vi "To-do-list-Labview.vi"() -> ()   [LabVIEW 2022 SP3]
uses:
  <vilib>/addons/database/Connection.llb/DB Tools Open Connec (String).vi
  <vilib>/addons/database/Connection.llb/Conn Execute.vi
  <vilib>/addons/database/Recordset.llb/Rec Destroy - Connection.vi
  <vilib>/addons/database/NI_Database_API.lvlib
panel:
  in  "TOT":bool
  in  "Afisare":bool
  in  "Calendar":timestamp=timestamp(3755242155.0327334 s since 1904-01-01) format="%<%x>T"
  in  "Efectuat":bool
  in  "Actualizare":bool
  in  "Stergere":bool
  in  "Editare":string
  in  "Sarcina de inserat":string
  in  "Inserare":bool
  in  "Alege linia":u16(ring) items=["1", "2", "4", "5", "9", "10", "11", "12", "14", "15", "16", "17"]
  out "Linii":i32
  out "Coloane":i32
  out "Lista de sarcini":string[][](table)
  # "Proiectul de fata are scopul de a facilita utilizatorului o metoda de a stoca, citii, edita, sterge informatii pe care le doreste. \n    Cu alte cuvinte, proiectul este un ToDoList in care, cu operatii de tip CRUD, se pot accesa datele dintr-o baza de date, iar utilizatorul are acces total la informatiile pe care acesta le introduce.\n     Ca si baza de date am ales Microsoft MySQL ce permite cu usurinta administratorilor sa acceseze datele in baze de date."
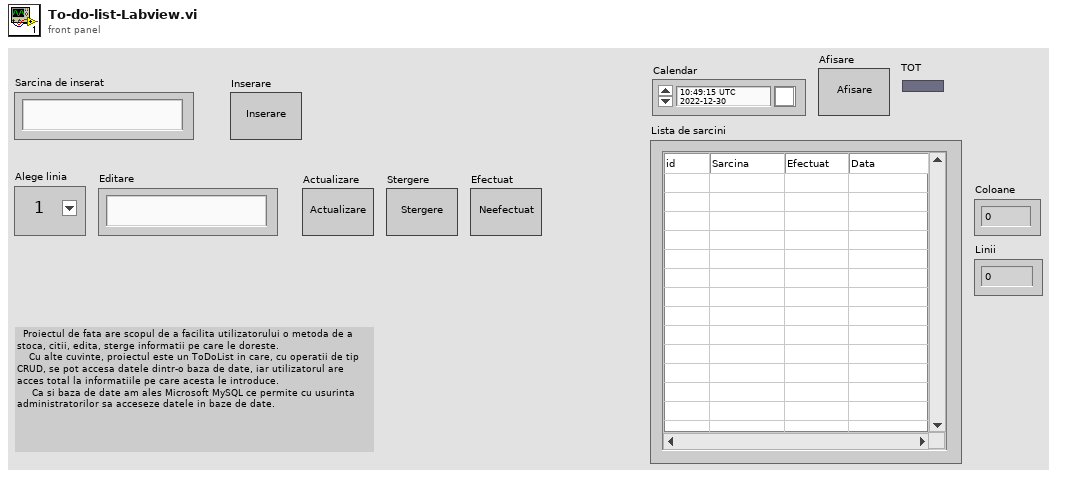
[diagram p1: front panel]
types:
  T1 = typedef "NI_Database_API.lvlib/Conn ObjectReference.ctl" = refnum<k1>
  T2 = typedef "NI_Database_API.lvlib/Rec ObjectReference.ctl" = refnum<k1>
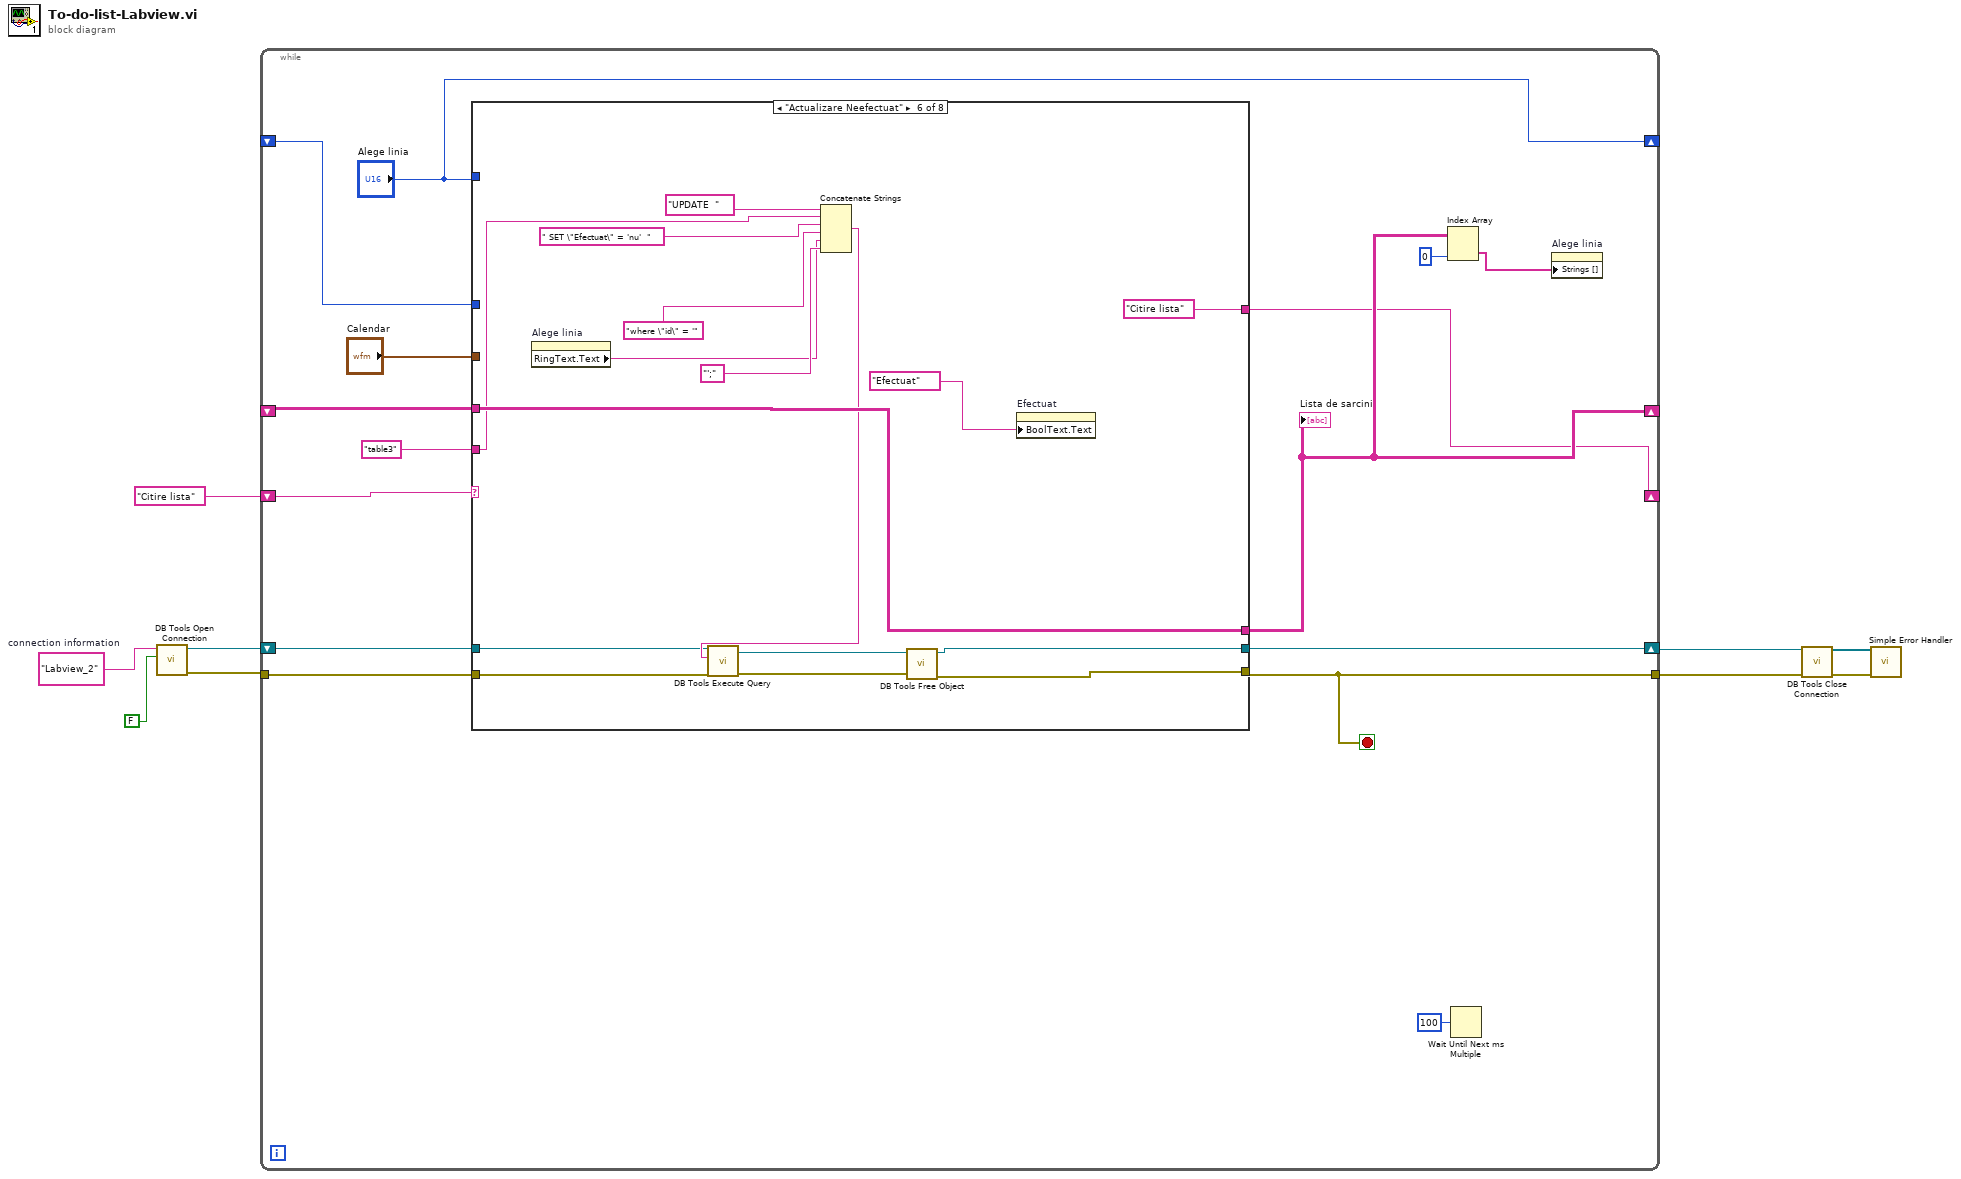
[diagram p0: block diagram]
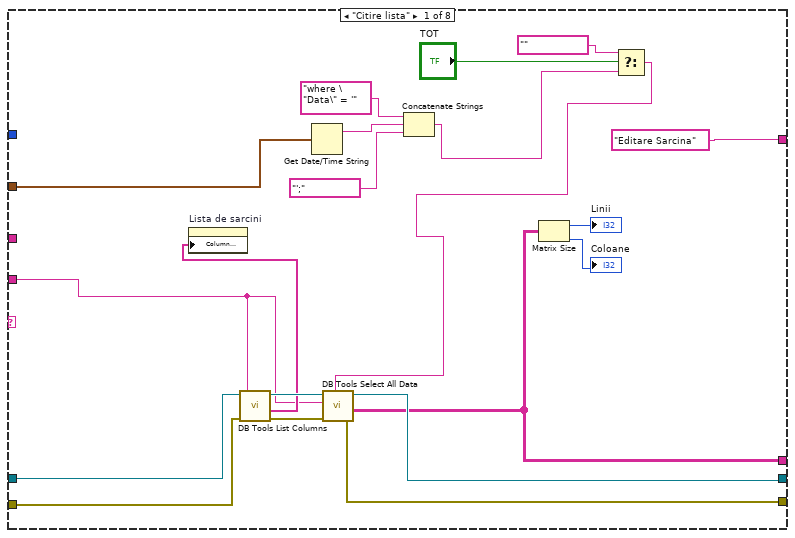
[diagram p2: hidden frame]
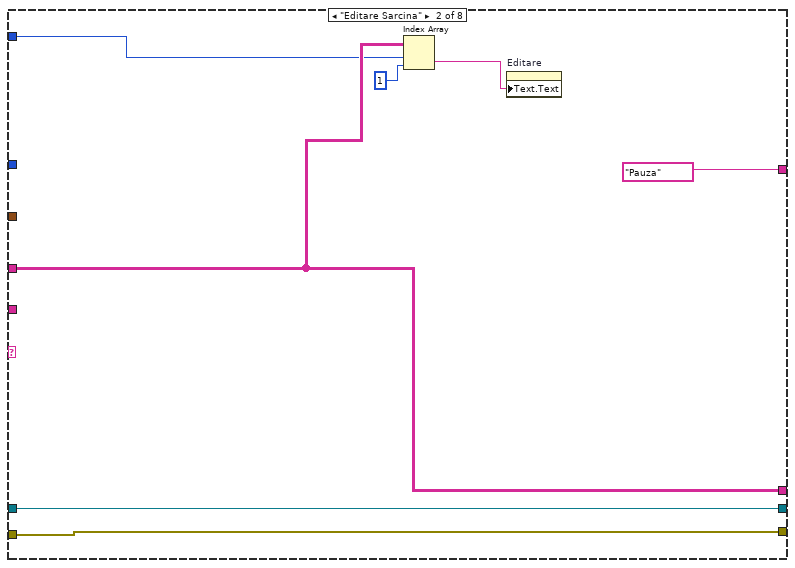
[diagram p3: hidden frame]
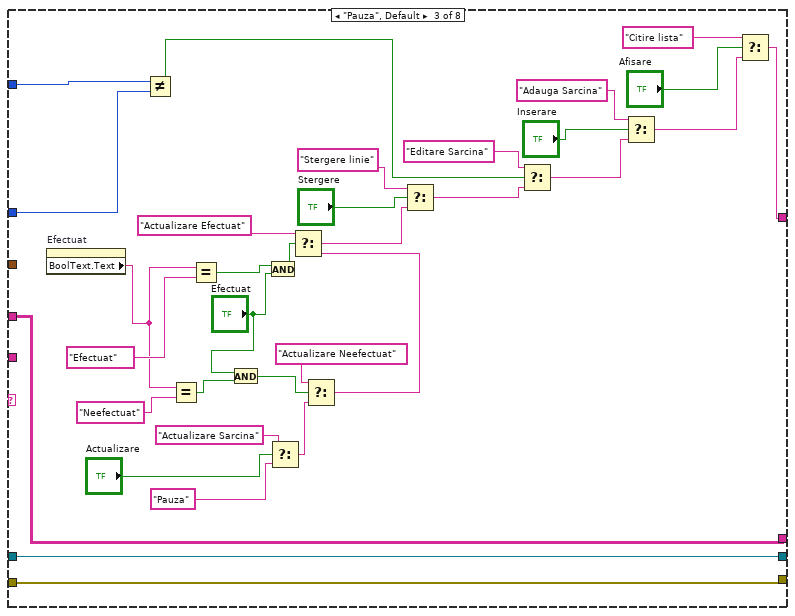
[diagram p4: hidden frame]
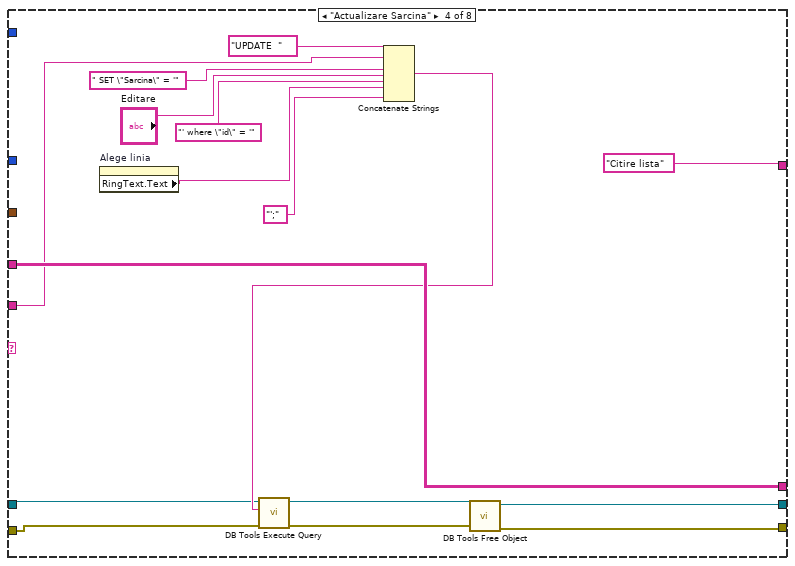
[diagram p5: hidden frame]
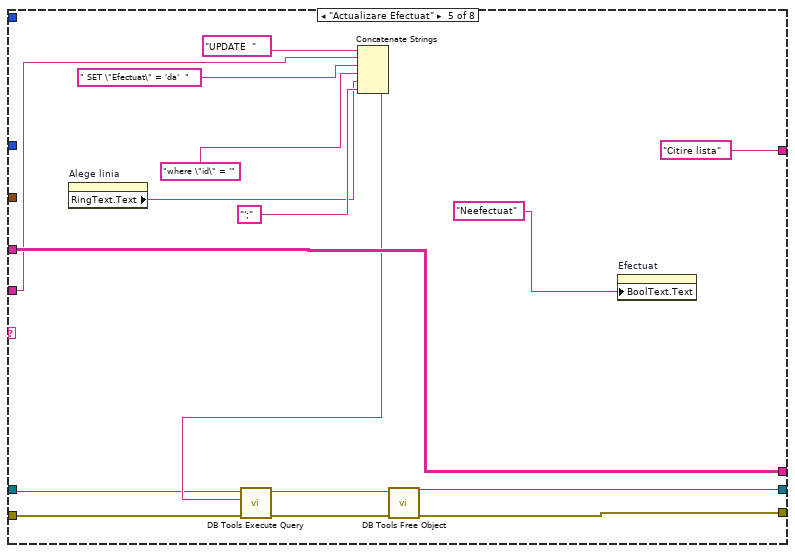
[diagram p6: hidden frame]
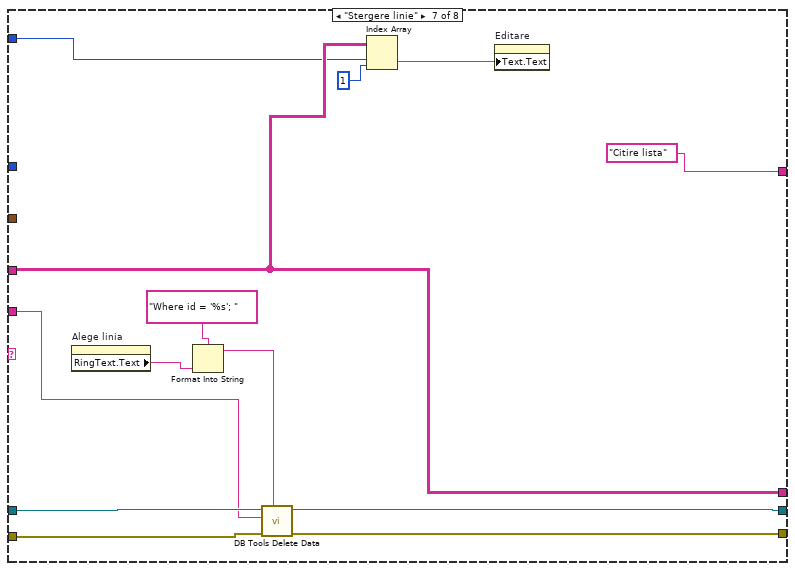
[diagram p7: hidden frame]
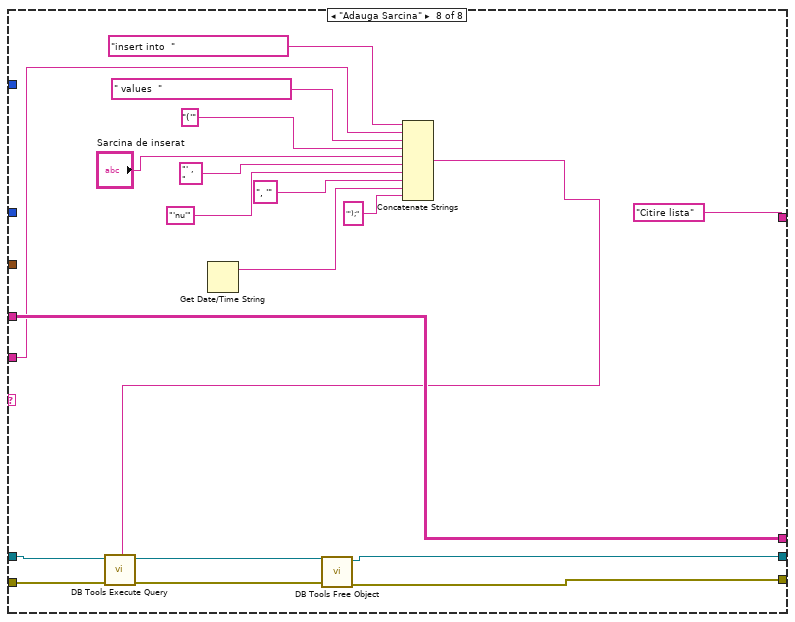
[diagram p8: hidden frame]
diagram:
  w8 = "Labview_2"  # connection information
  n1 = call-poly <vilib>:"DB Tools Open Connection.vi"("prompt? (F)"=FALSE, "connection information"=w8) -> ("error out"=w6:errorcluster, "connection reference"=w7:T1)  [unwired: 6 in]
  n2 = while {
    shift-right: [w20] -> w3
    shift-left: w7 -> [w22]
    tunnel: w6 -> [w23]
    tunnel: [w21] -> w4
    shift-right: [w9] -> _
    shift-left: "Citire lista" -> [w19]
    shift-right: [w14] -> _
    shift-left: _ -> [w17]
    shift-right: ["Alege linia"] -> _
    shift-left: _ -> [w12]
    stop <- w21 stop-if-true
    n3 = case shown="\"Actualizare Neefectuat\"" w19 {
      tunnel: w23 -> [w35 w49 w80 w86 w106 w121 w141 w161]
      tunnel: w22 -> [w37 w50 w81 w89 w104 w117 w143 w148]
      tunnel: [w41 w49 w80 w84 w102 w119 w140 w145] -> w21
      tunnel: [w40 w50 w81 w87 w100 w116 w142 w147] -> w20
      tunnel: ["Editare Sarcina" "Pauza" w82 "Citire lista" "Citire lista" "Citire lista" "Citire lista" "Citire lista"] -> w9
      tunnel: [w38 w46 w79 w98 w114 w130 w135 w162] -> w14
      tunnel: w17 -> [_ w46 w79 w98 w114 w130 w135 w162]
      tunnel: "Alege linia" -> [_ w44 w74 _ _ _ w134 _]
      tunnel: w12 -> [_ _ w73 _ _ _ _ _]
      tunnel: "table3" ("table") -> [w32 _ _ w96 w112 w128 w132 w151]
      tunnel: "Calendar" -> [w31 _ _ _ _ _ _ _]
      frame "Citire lista" {
        n4 = call <vilib>:"DB Tools List Columns.vi"("error in (no error)"=w35, "table"=w32, "connection reference"=w37) -> ("error out"=w34:errorcluster, "columns"=w33:string[], "connection reference out"=w36:T1)  [unwired: 1 in, 1 out]
        n5 = property on="Lista de sarcini" class="Tbl (strict)"("Column Headers[]"=w33) -> ()  [unwired: 2 in, 2 out]
        n6 = Get Date/Time String(seconds (now)=w31) -> (date string=w29:string)  [unwired: 2 in, 1 out]
        n7 = Concatenate Strings("where \"Data\" = '", w29, "';") -> (w25:string)
        n8 = Select(t="", s="TOT", f=w25) -> (s? t:f=w27:string)
        n9 = call <vilib>:"DB Tools Select All Data.vi"("optional clause"=w27, "error in (no error)"=w34, "table"=w32, "connection reference"=w36) -> ("error out"=w41:errorcluster, "data"=w38:string[][], "connection reference out"=w40:T1)  [unwired: 2 in]
        n10 = Matrix Size(0:w38) -> (1:→"Linii":i32, 2:→"Coloane":i32)
      }
      frame "Editare Sarcina" {
        n11 = Index Array(array=w46, index (row)=w44, index (col)=1) -> (element=w45:string)
        n12 = property on="Editare" class="Str"("Text.Text"=w45) -> ()  [unwired: 2 in, 2 out]
      }
      frame "Pauza", Default {
        n13 = property on="Efectuat" class="Bool"() -> ("BoolText.Text"=w63:string)  [unwired: 2 in, 2 out]
        n14 = Not Equal?(x=w74, y=w73) -> (x != y?=w72:bool)
        n15 = Equal?(x=w63, y="Neefectuat") -> (x = y?=w56:bool)
        n16 = Equal?(x=w63, y="Efectuat") -> (x = y?=w59:bool)
        n17 = And(x="Efectuat", y=w56) -> (x .and. y?=w55:bool)
        n18 = And(x=w59, y="Efectuat") -> (x .and. y?=w58:bool)
        n19 = Select(t="Actualizare Sarcina", s="Actualizare", f="Pauza") -> (s? t:f=w54:string)
        n20 = Select(t="Actualizare Neefectuat", s=w55, f=w54) -> (s? t:f=w61:string)
        n21 = Select(t="Actualizare Efectuat", s=w58, f=w61) -> (s? t:f=w66:string)
        n22 = Select(t="Stergere linie", s="Stergere", f=w66) -> (s? t:f=w65:string)
        n23 = Select(t="Editare Sarcina", s=w72, f=w65) -> (s? t:f=w76:string)
        n24 = Select(t="Adauga Sarcina", s="Inserare", f=w76) -> (s? t:f=w77:string)
        n25 = Select(t="Citire lista", s="Afisare", f=w77) -> (s? t:f=w82:string)
      }
      frame "Actualizare Sarcina" {
        n26 = property on="Alege linia" class="Ring (strict)"() -> ("RingText.Text"=w92:string)  [unwired: 2 in, 2 out]
        n27 = Concatenate Strings("UPDATE  " ("table"), w96, " SET \"Sarcina\" = '" ("table"), "Editare", "' where \"id\" = '" ("table"), w92, "';" ("table")) -> (w90:string)
        n28 = call-poly <vilib>:"DB Tools Execute Query.vi"("error in (no error)"=w86, "SQL query"=w90, "connection reference"=w89) -> ("error out"=w85:errorcluster, "recordset reference"=w88:T2)  [unwired: 5 in]
        n29 = call-poly <vilib>:"DB Tools Free Object.vi"("error in (no error)"=w85, "recordset reference"=w88) -> ("error out"=w84:errorcluster, "connection reference"=w87:T1)  [unwired: 8 in]
      }
      frame "Actualizare Efectuat" {
        n30 = property on="Alege linia" class="Ring (strict)"() -> ("RingText.Text"=w108:string)  [unwired: 2 in, 2 out]
        n31 = Concatenate Strings("UPDATE  " ("table"), w112, " SET \"Efectuat\" = 'da'  " ("table"), "where \"id\" = '" ("table"), w108, "';" ("table")) -> (w105:string)
        n32 = call-poly <vilib>:"DB Tools Execute Query.vi"("error in (no error)"=w106, "SQL query"=w105, "connection reference"=w104) -> ("error out"=w101:errorcluster, "recordset reference"=w103:T2)  [unwired: 5 in]
        n33 = call-poly <vilib>:"DB Tools Free Object.vi"("error in (no error)"=w101, "recordset reference"=w103) -> ("error out"=w102:errorcluster, "connection reference"=w100:T1)  [unwired: 8 in]
        n34 = property on="Efectuat" class="Bool"("BoolText.Text"="Neefectuat") -> ()  [unwired: 2 in, 2 out]
      }
      frame "Actualizare Neefectuat" {
        n35 = property on="Alege linia" class="Ring (strict)"() -> ("RingText.Text"=w123:string)  [unwired: 2 in, 2 out]
        n36 = Concatenate Strings("UPDATE  " ("table"), w128, " SET \"Efectuat\" = 'nu'  " ("table"), "where \"id\" = '" ("table"), w123, "';" ("table")) -> (w124:string)
        n37 = call-poly <vilib>:"DB Tools Execute Query.vi"("error in (no error)"=w121, "SQL query"=w124, "connection reference"=w117) -> ("error out"=w120:errorcluster, "recordset reference"=w118:T2)  [unwired: 5 in]
        n38 = call-poly <vilib>:"DB Tools Free Object.vi"("error in (no error)"=w120, "recordset reference"=w118) -> ("error out"=w119:errorcluster, "connection reference"=w116:T1)  [unwired: 8 in]
        n39 = property on="Efectuat" class="Bool"("BoolText.Text"="Efectuat") -> ()  [unwired: 2 in, 2 out]
      }
      frame "Stergere linie" {
        n40 = property on="Alege linia" class="Ring (strict)"() -> ("RingText.Text"=w139:string)  [unwired: 2 in, 2 out]
        n41 = Format Into String(format string="Where id = '%s'; " ("table"), w139) -> (resulting string=w137:string)  [unwired: 2 in, 1 out]
        n42 = call <vilib>:"DB Tools Delete Data.vi"("condition"=w137, "error in (no error)"=w141, "table"=w132, "connection reference"=w143) -> ("error out"=w140:errorcluster, "connection reference out"=w142:T1)  [unwired: 6 in]
        n43 = Index Array(array=w135, index (row)=w134, index (col)=1) -> (element=w133:string)
        n44 = property on="Editare" class="Str"("Text.Text"=w133) -> ()  [unwired: 2 in, 2 out]
      }
      frame "Adauga Sarcina" {
        n45 = Get Date/Time String() -> (date string=w155:string)  [unwired: 3 in, 1 out]
        n46 = Concatenate Strings("insert into  " ("table"), w151, " values  " ("table"), "('" ("table"), "Sarcina de inserat", "' , " ("table"), "'nu'" ("table"), ", '" ("table"), w155, "');" ("table")) -> (w150:string)
        n47 = call-poly <vilib>:"DB Tools Execute Query.vi"("error in (no error)"=w161, "SQL query"=w150, "connection reference"=w148) -> ("error out"=w146:errorcluster, "recordset reference"=w149:T2)  [unwired: 5 in]
        n48 = call-poly <vilib>:"DB Tools Free Object.vi"("error in (no error)"=w146, "recordset reference"=w149) -> ("error out"=w145:errorcluster, "connection reference"=w147:T1)  [unwired: 8 in]
      }
    }
    "Lista de sarcini" <- w14
    n49 = Index Array(array=w14, index (col)=0 ("index")) -> (element=w16:string[])  [unwired: 1 in]
    n50 = Wait Until Next ms Multiple(millisecond multiple=u32 100) -> ()  [unwired: 1 out]
    n51 = property on="Alege linia" class="Ring (strict)"("Strings []"=w16) -> ()  [unwired: 2 in, 2 out]
  }
  n52 = call <vilib>:"DB Tools Close Connection.vi"("error in (no error)"=w4, "connection reference"=w3) -> ("error out"=w5:errorcluster)  [unwired: 5 in]
  n53 = call <vilib>:"Simple Error Handler.vi"("error in (no error)"=w5) -> ()  [unwired: 4 in, 5 out]
